vi "seq_delay_PB.vi"(7 "delay(ns)":dbl[](array[numeric])=[0.0, 298.0, 875.0, 0.0, 0.0, 0.0, 298.0], 11 "PB Instructions":T1[](array[typedef])=[{"Instr. Data"=0, "Op Code"=enum."Continue", "Flags"=[TRUE, FALSE, FALSE, FALSE, FALSE, FALSE, FALSE, FALSE, FALSE, FALSE, FALSE, FALSE, FALSE, FALSE, FALSE, FALSE, FALSE, FALSE, FALSE, FALSE, FALSE, FALSE, FALSE, FALSE], "Comments"="tau", "Time"=5e-08}, {"Instr. Data"=0, "Op Code"=enum."Continue", "Flags"=[FALSE, FALSE, TRUE, FALSE, FALSE, FALSE, FALSE, FALSE, FALSE, FALSE, FALSE, FALSE, FALSE, FALSE, FALSE, FALSE, FALSE, FALSE, FALSE, FALSE, FALSE, FALSE, FALSE, FALSE], "Comments"="", "Time"=5e-09}, {"Instr. Data"=0, "Op Code"=enum."Continue", "Flags"=[FALSE, FALSE, FALSE, FALSE, FALSE, FALSE, FALSE, FALSE, FALSE, FALSE, FALSE, FALSE, FALSE, FALSE, FALSE, FALSE, FALSE, FALSE, FALSE, FALSE, FALSE, FALSE, FALSE, FALSE], "Comments"="", "Time"=4.5e-08}, {"Instr. Data"=0, "Op Code"=enum."Continue", "Flags"=[FALSE, FALSE, TRUE, FALSE, FALSE, FALSE, FALSE, FALSE, FALSE, FALSE, FALSE, FALSE, FALSE, FALSE, FALSE, FALSE, FALSE, FALSE, FALSE, FALSE, FALSE, FALSE, FALSE, FALSE], "Comments"="", "Time"=5e-09}, {"Instr. Data"=0, "Op Code"=enum."Continue", "Flags"=[FALSE, FALSE, FALSE, FALSE, FALSE, FALSE, FALSE, FALSE, FALSE, FALSE, FALSE, FALSE, FALSE, FALSE, FALSE, FALSE, FALSE, FALSE, FALSE, FALSE, FALSE, FALSE, FALSE, FALSE], "Comments"="", "Time"=2e-06}] {"Time" format="%#.3p"}) -> (3 "PB Instructions output":T1[](array[typedef])=[{"Instr. Data"=0, "Op Code"=enum."Continue", "Flags"=[TRUE, FALSE, FALSE, FALSE, FALSE, FALSE, FALSE, FALSE], "Comments"="", "Time"=5e-08}, {"Instr. Data"=0, "Op Code"=enum."Continue", "Flags"=[FALSE, FALSE, FALSE, FALSE, FALSE, FALSE, FALSE, FALSE], "Comments"="", "Time"=8.789999999999999e-07}, {"Instr. Data"=0, "Op Code"=enum."Continue", "Flags"=[FALSE, FALSE, TRUE, FALSE, FALSE, FALSE, FALSE, FALSE], "Comments"="", "Time"=5e-09}, {"Instr. Data"=0, "Op Code"=enum."Continue", "Flags"=[FALSE, FALSE, FALSE, FALSE, FALSE, FALSE, FALSE, FALSE], "Comments"="", "Time"=4.5e-08}, {"Instr. Data"=0, "Op Code"=enum."Continue", "Flags"=[FALSE, FALSE, TRUE, FALSE, FALSE, FALSE, FALSE, FALSE], "Comments"="", "Time"=5e-09}, {"Instr. Data"=0, "Op Code"=enum."Continue", "Flags"=[FALSE, FALSE, FALSE, FALSE, FALSE, FALSE, FALSE, FALSE], "Comments"="", "Time"=2e-06}] {"Time" format="%#.3p"})   [LabVIEW 2020, in "SiC_Properties_Test.lvlib"]
uses:
  EP_SiC_Properties_Test/SiC_Properties_Test.lvlib
  HW_SpinCore_PB/SpinCore PulseBlaster/PB Instruction.ctl
  HW_SpinCore_PB/SpinCore PulseBlaster/SpinCore PulseBluster.lvlib
panel:
  out "time input":dbl[][](array[numeric])=[[0.0, 2.98e-07, 8.79e-07, 0.0, 0.0, 0.0, 2.98e-07], [5e-08, 5e-08, 5e-08, 5e-08, 5e-08, 5e-08, 5e-08], [5e-09, 5e-09, 5e-09, 5e-09, 5e-09, 5e-09, 5e-09], [4.5e-08, 4.5e-08, 4.5e-08, 4.5e-08, 4.5e-08, 4.5e-08, 4.5e-08], [5e-09, 5e-09, 5e-09, 5e-09, 5e-09, 5e-09, 5e-09], [2e-06, 2e-06, 2e-06, 2e-06, 2e-06, 2e-06, 2e-06], [8.79e-07, 5.81e-07, 0.0, 8.79e-07, 8.79e-07, 8.79e-07, 5.81e-07]]
  out "time sequece after adding delay":dbl[](array[numeric])=[5e-08, 5e-09, 4.5e-08, 5e-09, 1.93e-07, 5e-08, 5e-09, 4.5e-08, 5e-09, 4.7600000000000013e-07, 5e-08, 5e-09, 4.5e-08, 5e-09, 1.121e-06, 2.9799999999999994e-07, 5.81e-07, 0.0, 0.0]
  out "operation sequece after adding delay":dbl[][](array[numeric])=[[1.0, 0.0, 0.0, 0.0, 0.0, 0.0, 0.0], [0.0, 0.0, 0.0, 0.0, 0.0, 0.0, 0.0], [0.0, 0.0, 0.0, 0.0, 0.0, 0.0, 0.0], [0.0, 0.0, 0.0, 0.0, 0.0, 0.0, 0.0], [0.0, 0.0, 0.0, 0.0, 0.0, 0.0, 0.0], [0.0, 0.0, 0.0, 0.0, 0.0, 0.0, 0.0], [0.0, 0.0, 0.0, 0.0, 0.0, 0.0, 0.0], [0.0, 0.0, 0.0, 0.0, 0.0, 0.0, 0.0], [0.0, 0.0, 0.0, 0.0, 0.0, 0.0, 0.0], [0.0, 0.0, 0.0, 0.0, 0.0, 0.0, 0.0], [0.0, 0.0, 0.0, 0.0, 0.0, 0.0, 0.0], [0.0, 0.0, 1.0, 0.0, 0.0, 0.0, 0.0], [0.0, 0.0, 0.0, 0.0, 0.0, 0.0, 0.0], [0.0, 0.0, 1.0, 0.0, 0.0, 0.0, 0.0], [0.0, 0.0, 0.0, 0.0, 0.0, 0.0, 0.0], [0.0, 0.0, 0.0, 0.0, 0.0, 0.0, 0.0], [0.0, 0.0, 0.0, 0.0, 0.0, 0.0, 0.0], [0.0, 0.0, 0.0, 0.0, 0.0, 0.0, 0.0], [0.0, 0.0, 0.0, 0.0, 0.0, 0.0, 0.0]]
  out "time seq_ol":dbl[](array[numeric])=[5e-08, 8.789999999999999e-07, 5e-09, 4.5e-08, 5e-09, 2e-06]
  out "oper_sol":dbl[][](array[numeric])=[[1.0, 0.0, 0.0, 0.0, 0.0, 0.0, 0.0], [0.0, 0.0, 0.0, 0.0, 0.0, 0.0, 0.0], [0.0, 0.0, 1.0, 0.0, 0.0, 0.0, 0.0], [0.0, 0.0, 0.0, 0.0, 0.0, 0.0, 0.0], [0.0, 0.0, 1.0, 0.0, 0.0, 0.0, 0.0], [0.0, 0.0, 0.0, 0.0, 0.0, 0.0, 0.0]]
  out "opprator array":dbl[][](array[numeric])=[[0.0, 0.0, 0.0, 0.0, 0.0, 0.0, 0.0], [1.0, 0.0, 0.0, 0.0, 0.0, 0.0, 0.0], [0.0, 0.0, 1.0, 0.0, 0.0, 0.0, 0.0], [0.0, 0.0, 0.0, 0.0, 0.0, 0.0, 0.0], [0.0, 0.0, 1.0, 0.0, 0.0, 0.0, 0.0], [0.0, 0.0, 0.0, 0.0, 0.0, 0.0, 0.0], [0.0, 0.0, 0.0, 0.0, 0.0, 0.0, 0.0]]
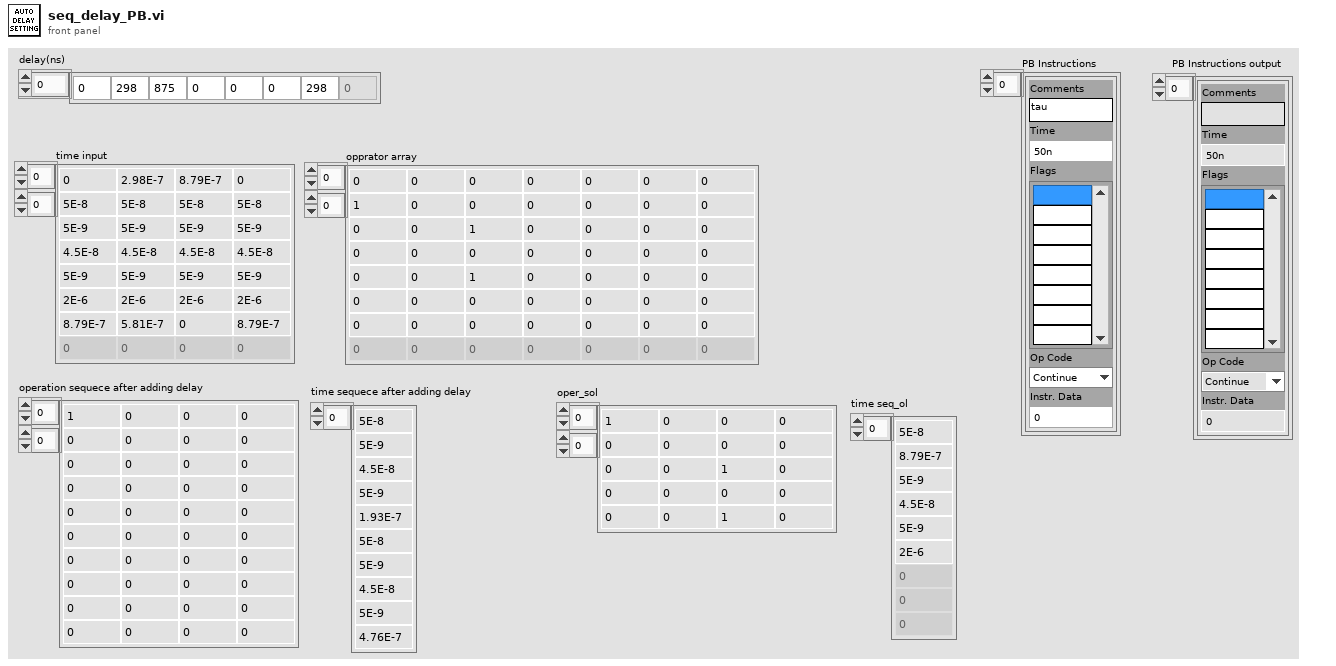
[diagram p1: front panel]
types:
  T1 = typedef "SpinCore PulseBluster.lvlib/PB Instruction.ctl" = cluster{"Instr. Data":i32, "Op Code":enum16{"Continue", "Stop", "Loop", "End Loop", "JSR", "RTS", "Branch", "Long Delay", "Wait"}, "Flags":bool[], "Comments":string, "Time":dbl}
  T2 = enum16{"Continue", "Stop", "Loop", "End Loop", "JSR", "RTS", "Branch", "Long Delay", "Wait"}
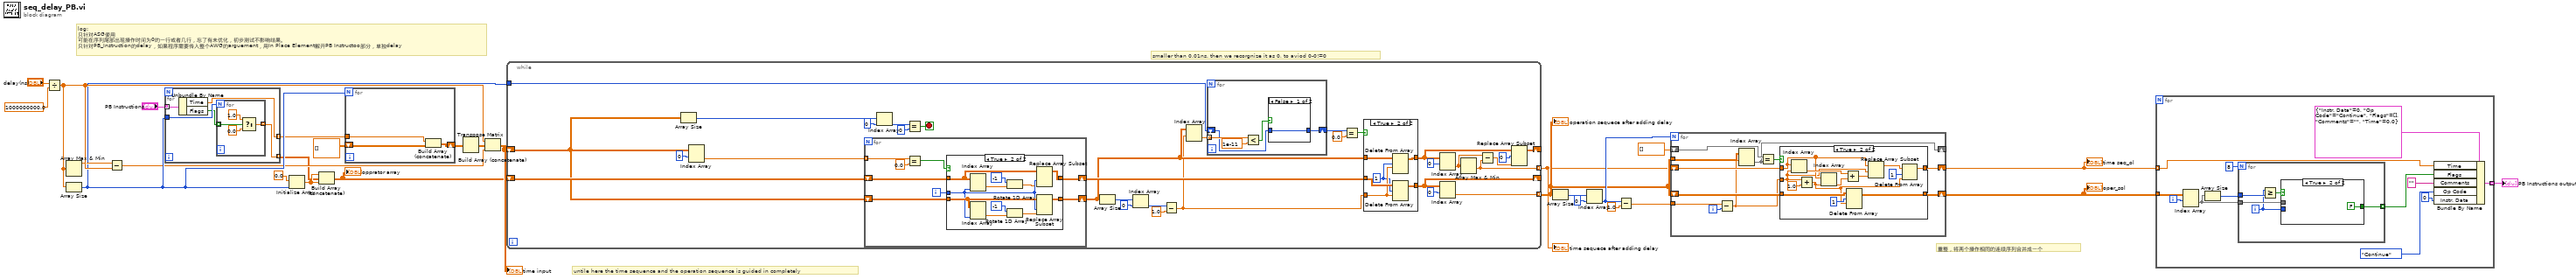
[diagram p0: block diagram]
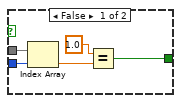
[diagram p3: hidden frame]
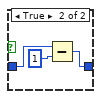
[diagram p4: hidden frame]
diagram:
  # "log:\n只针对ASG使用\n可能在序列尾部出现操作时间为0的一行或者几行，忘了有未优化，初步测试不影响结果。\n只针对PB_Instruction的delay，如果程序需要传入整个AWG的arguement，用In Place Element解开PB Instructoo部分，单独delay"
  # "untile here the time sequence and the operation sequence is guided in completely"
  # "重整，将两个操作相同的连续序列合并成一个"
  # "smaller than 0.01ns. then we recorgnize it as 0, to aviod 0-0!=0"
  n1 = Divide(x="delay(ns)", y=1000000000.0 ("Numeric")) -> (x/y=w25:dbl[])
  n2 = Array Max & Min(array=w25) -> (max value=w18:dbl)  [unwired: 3 out]
  n3 = Array Size(array=w25) -> (size(s)=w16:i32)
  n4 = Subtract(x=w18, y=w25) -> (x-y=w14:dbl[])
  n5 = for {
    tunnel: "PB Instructions" -> [w32] mode=indexing
    tunnel: w16 -> [w31]
    tunnel: [w30] -> w9 mode=indexing
    tunnel: [w29] -> w10 mode=indexing
    n6 = Unbundle By Name(w32) -> ("Time"=w29:dbl, "Flags"=w28:bool[])
    n7 = for {
      N: w31 -> [_]
      tunnel: w28 -> [w36] mode=indexing
      tunnel: [w33] -> w30 mode=indexing
      n8 = Select(t=1.0, s=w36, f=0.0) -> (s? t:f=w33:dbl)
    }
  }
  n9 = Initialize Array(0.0 ("element"), w16) -> (w12:dbl[])
  n10 = Build Array (concatenate)(w12, w9, w12) -> (w15:dbl[][])
  "opprator array" <- w15
  n11 = for {
    N: w16 -> [_]
    tunnel: w10 -> [w39]
    shift-right: [w38] -> w11
    shift-left: dbl[][] [] -> [w37]
    n12 = Build Array (concatenate)(w39, w37) -> (w38:dbl[][])
  }
  n13 = Transpose Matrix(1:w11) -> (0:w13:dbl[][])
  n14 = Build Array (concatenate)(w25, w13, w14) -> (w17:dbl[][])
  "time input" <- w17
  n15 = while {
    tunnel: w16 -> [w44]
    tunnel: [w62] -> w19 mode=indexing
    tunnel: [w60] -> w21 mode=indexing
    shift-right: [w51] -> _
    shift-left: w17 -> [w53]
    shift-right: [w59] -> _
    shift-left: w15 -> [w69]
    stop <- w54 stop-if-true
    n16 = Array Size(array=w53) -> (size(s)=w57:i32[])
    n17 = Index Array(array=w53, index (row)=0) -> (element=w68:dbl[])  [unwired: 1 in]
    n18 = for {
      tunnel: w68 -> [w91] mode=indexing
      shift-right: [w92] -> w49
      shift-left: w53 -> [w93]
      shift-right: [w90] -> w67
      shift-left: w69 -> [w88]
      i -> [w89]
      n19 = Equal?(x=w91, y=0.0) -> (x = y?=w94:bool)
      n20 = case shown="True" w94 {
        tunnel: w93 -> [w97 w104]
        tunnel: w89 -> [_ w101]
        tunnel: w88 -> [w96 w102]
        tunnel: [w97 w99] -> w92
        tunnel: [w96 w98] -> w90
        frame False {
        }
        frame True {
          n21 = Index Array(array=w102, index (col)=w101) -> (element=w105:dbl[])  [unwired: 1 in]
          n22 = Index Array(array=w104, index (col)=w101) -> (element=w108:dbl[])  [unwired: 1 in]
          n23 = Rotate 1D Array(1:w105, 2:-1 ("n")) -> (0:w100:dbl[])
          n24 = Rotate 1D Array(1:w108, 2:-1 ("n")) -> (0:w103:dbl[])
          n25 = Replace Array Subset(array=w102, new element=w100, index (col)=w101) -> (w98:dbl[][])  [unwired: 1 in]
          n26 = Replace Array Subset(array=w104, new element=w103, index (col)=w101) -> (w99:dbl[][])  [unwired: 1 in]
        }
      }
    }
    n27 = Index Array(array=w57, index=0) -> (element=w56:i32)
    n28 = Equal?(x=w56, y=0) -> (x = y?=w54:bool)
    n29 = Array Size(array=w49) -> (size(s)=w48:i32[])
    n30 = Index Array(array=w48, index=0) -> (element=w45:i32)
    n31 = Subtract(x=w45, y=1.0) -> (x-y=w40:dbl)
    n32 = Index Array(array=w49, index (row)=w40) -> (element=w50:dbl[])  [unwired: 1 in]
    n33 = for {
      tunnel: w50 -> [w75] mode=indexing
      shift-right: [w71] -> w41
      shift-left: w44 -> [w72]
      n34 = Less?(x=w75, y=1e-11) -> (x < y?=w73:bool)
      n35 = case shown="False" w73 {
        tunnel: w72 -> [w76 w79]
        tunnel: [w76 w77] -> w71
        frame False {
        }
        frame True {
          n36 = Subtract(x=w79, y=1) -> (x-y=w77:i32)
        }
      }
    }
    n37 = Equal?(x=w41, y=0.0) -> (x = y?=w42:bool)
    n38 = case shown="True" w42 {
      tunnel: w49 -> [w80 w87]
      tunnel: [w80 w86] -> w65
      tunnel: w67 -> [w81 w84]
      tunnel: [w81 w85] -> w59
      tunnel: w40 -> [_ w83]
      frame False {
      }
      frame True {
        w82 = 1 ("length")
        n39 = Delete From Array(array=w87, length=w82, index (row)=w83) -> (array with subset deleted=w86:dbl[][])  [unwired: 1 in, 1 out]
        n40 = Delete From Array(array=w84, length=w82, index (row)=w83) -> (array with subset deleted=w85:dbl[][])  [unwired: 1 in, 1 out]
      }
    }
    n41 = Index Array(array=w65, index (row)=0) -> (element=w63:dbl[])  [unwired: 1 in]
    n42 = Index Array(array=w59, index (row)=0) -> (element=w60:dbl[])  [unwired: 1 in]
    n43 = Array Max & Min(array=w63) -> (min value=w62:dbl)  [unwired: 3 out]
    n44 = Subtract(x=w63, y=w62) -> (x-y=w64:dbl[])
    n45 = Replace Array Subset(array=w65, new element=w64, index (row)=0) -> (w51:dbl[][])  [unwired: 1 in]
  }
  "time sequece after adding delay" <- w19
  "operation sequece after adding delay" <- w21
  n46 = Array Size(array=w21) -> (size(s)=w22:i32[])
  n47 = Index Array(array=w22, index=0) -> (element=w24:i32)
  n48 = Subtract(x=w24, y=1.0) -> (x-y=w23:dbl)
  n49 = for {
    N: w24 -> [_]
    tunnel: w21 -> [w113]
    shift-right: [w112] -> _
    shift-left: dbl[] [] -> [w118]
    shift-right: [w114] -> w20
    shift-left: w21 -> [w117]
    shift-right: [w115] -> w27
    shift-left: w19 -> [w116]
    tunnel: w23 -> [w110]
    i -> [w111]
    n50 = Subtract(x=w110, y=w111) -> (x-y=w109:dbl)
    n51 = Index Array(array=w113, index (row)=w109) -> (element=w112:dbl[])  [unwired: 1 in]
    n52 = Equal?(x=w118, y=w112) -> (x = y?=w119:bool)
    n53 = case shown="True" w119 {
      tunnel: w109 -> [_ w124]
      tunnel: w117 -> [w120 w134]
      tunnel: [w120 w133] -> w114
      tunnel: w116 -> [w121 w129]
      tunnel: [w121 w126] -> w115
      frame False {
      }
      frame True {
        n54 = Index Array(array=w129, index=w124) -> (element=w131:dbl)
        n55 = Add(x=w124, y=1.0) -> (x+y=w122:dbl)
        n56 = Index Array(array=w129, index=w122) -> (element=w132:dbl)
        n57 = Add(x=w131, y=w132) -> (x+y=w130:dbl)
        n58 = Delete From Array(array=w134, length=1, index (row)=w122) -> (array with subset deleted=w133:dbl[][])  [unwired: 1 in, 1 out]
        n59 = Replace Array Subset(array=w129, new element=w130, index=w124) -> (w128:dbl[])
        n60 = Delete From Array(array=w128, length=1, index=w122) -> (array with subset deleted=w126:dbl[])  [unwired: 1 out]
      }
    }
  }
  "time seq_ol" <- w27
  "oper_sol" <- w20
  n61 = for {
    tunnel: w20 -> [w146]
    tunnel: [w138] -> w1 mode=indexing
    tunnel: w27 -> [w140] mode=indexing
    i -> [w144]
    n62 = Index Array(array=w146, index (row)=w144) -> (element=w145:dbl[])  [unwired: 1 in]
    n63 = Array Size(array=w145) -> (size(s)=w135:i32)
    n64 = for {
      N: 8 -> [_]
      tunnel: w145 -> [w151]
      tunnel: [w147] -> w139 mode=indexing
      tunnel: w135 -> [w149]
      i -> [w148]
      n65 = Greater Or Equal?(x=w148, y=w149) -> (x >= y?=w150:bool)
      n66 = case shown="True" w150 {
        tunnel: w151 -> [w155 _]
        tunnel: w148 -> [w153 _]
        tunnel: [w152 FALSE ("x = y?")] -> w147
        frame False {
          n67 = Index Array(array=w155, index=w153) -> (element=w154:dbl)
          n68 = Equal?(x=1.0, y=w154) -> (x = y?=w152:bool)
        }
        frame True {
        }
      }
    }
    n69 = Bundle By Name(cluster=T1 {"Instr. Data"=0, "Op Code"=enum."Continue", "Flags"=[], "Comments"="", "Time"=0.0} ("PB Instruction"), "Time"=w140, "Flags"=w139, "Comments"="", "Op Code"=T2."Continue", "Instr. Data"=0) -> (w138:T1)
  }
  "PB Instructions output" <- w1
